vi "Control Laser.vi"(8 "error in (no error)":errorcluster {"code" format="%.0x"}, 10 "State":bool, 11 "Device ID (0)":i32) -> (0 "error out":errorcluster {"code" format="%.0x"}, 3 "Device ID out":i32)   [LabVIEW 2020, in "KEYENCE LJ-X8000A.lvlib"]
doc: "This function permits/prohibits the emission of the laser."
uses:
  KEYENCE LJ-X8000A.lvlib
panel:
  # "(c) 2019 KEYENCE CORPORATION.  ALL RIGHTS RESERVED."
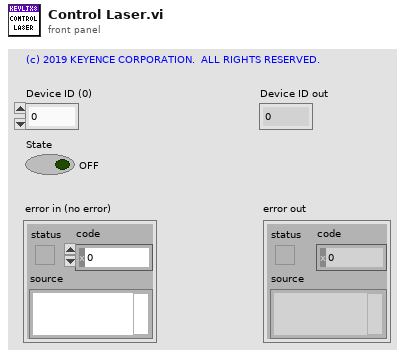
[diagram p1: front panel]
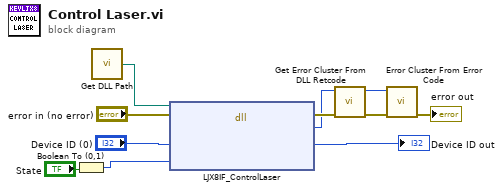
[diagram p0: block diagram]
diagram:
  n1 = Boolean To (0,1)(Boolean="State") -> (0, 1=w3:i16)
  n2 = call "Get DLL Path.vi"() -> ("DLL Path"=w8:path)  [unwired: 3 in]
  n3 = dll-call lib="C:/Program Files (x86)/National Instruments/LabVIEW 2018/instr.lib/KEYENCE LJ-X8000/LJX8_IF.*" fn="LJX8IF_ControlLaser"(path in=w8, error in="error in (no error)", "lDeviceId"="Device ID (0)", "byState"=w3) -> (error out=w6:errorcluster, "lRetCode"=w5:i32, "lDeviceId"=→"Device ID out":i32)  [unwired: 2 in, 1 out]
  n4 = call "Get Error Cluster From DLL Retcode.vi"("error in (no error)"=w6, "DLL Return Code"=w5) -> ("error out"=w7:errorcluster, "VI Error Code"=w1:i32)  [unwired: 8 in]
  n5 = call <vilib>:"Error Cluster From Error Code.vi"("error in (no error)"=w7, "error code (0)"=w1) -> ("error out"=→"error out":errorcluster)  [unwired: 7 in]
